vi "Read Attributes.vi"(11 "WebSocket Data Msg":refnum<class "WebSocket Data Handler Msg.lvclass">) -> (2 "Payload":cluster{"Data":string})   [LabVIEW 2016, in "WebSocket Actor.lvlib" / "WebSocket Data Handler Msg.lvclass"]
uses:
  WebSocket Data Handler Msg.lvclass
  WebSocket Data Handler Msg.lvclass/WebSocket Data Handler Msg.ctl
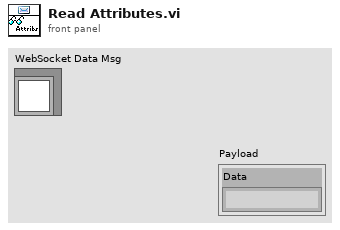
[diagram p1: front panel]
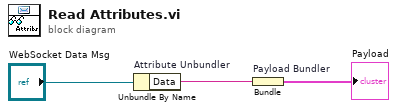
[diagram p0: block diagram]
diagram:
  n1 = Unbundle By Name "Attribute Unbundler"("WebSocket Data Msg") -> ("Data"=w1:string)
  n2 = Bundle "Payload Bundler"("Data"=w1) -> (→"Payload":cluster{"Data":string})  [unwired: 1 in]
